vi "Keysight E36300 Series Run Data Logger.vi"() -> ()   [LabVIEW 2020]
doc: "This example runs data logger.\n\nNote:\nThis VI is only available on the E36312A and E36313A models."
uses:
  Keysight E36300 Series.lvlib
panel:
  in  "Channel (1)":string="1"
  out "Logged Data":dbl[](array[numeric])
  in  "Reading Count (0)":i32
  in  "Trigger Source (0: Bus)":i32(ring) items=["Bus", "External", "Immediate"]
  in  "Sample Interval (0.2 sec)":dbl=0.2
  in  "Sample Duration (1 sec)":dbl=1.0
  in  "Enable Extremum (T: Enable)":bool=TRUE
  in  "Enable Data Logging (T: Enable)":bool=TRUE
  in  "Data Logging (0: Current)":i32(ring) items=["Current", "Voltage"]
  in  "Data Save Path(\"External:\\log_1.csv\")":string="\"External:\\log_1.csv\""
  in  "VISA resource name":refnum<visa-resource-name>
  # "(c) 2019 - 2021 National Instruments.  ALL RIGHTS RESERVED."
  # "This VI is only available on the E36312A and E36313A models."
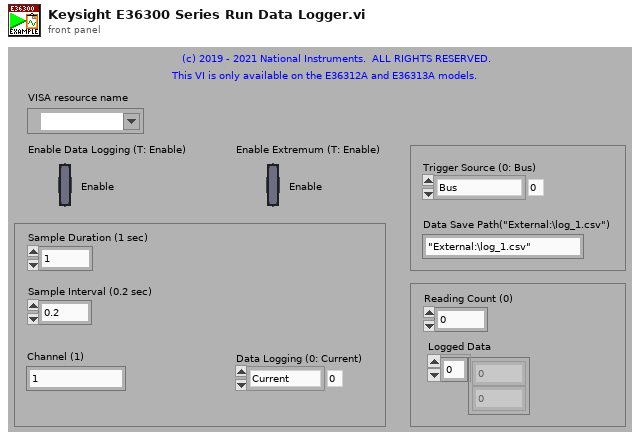
[diagram p1: front panel]
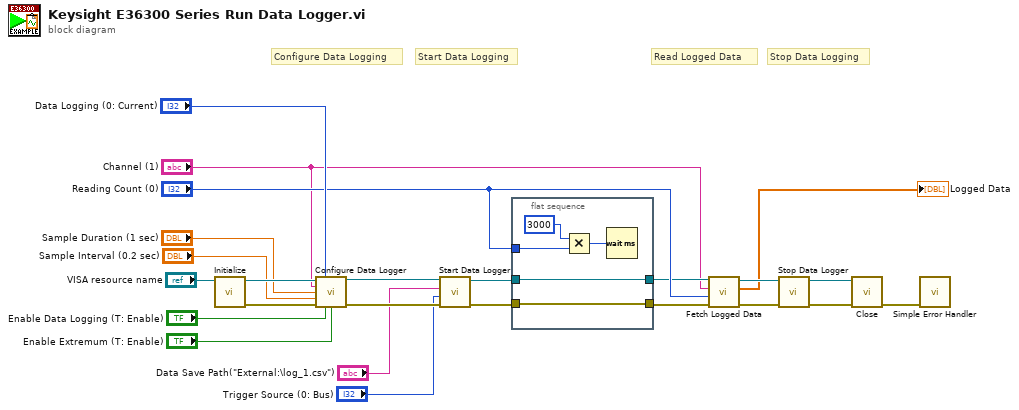
[diagram p0: block diagram]
diagram:
  # "Read Logged Data"
  # "Stop Data Logging"
  # "Start Data Logging"
  # "Configure Data Logging"
  n1 = call "Initialize.vi"("VISA resource name"="VISA resource name") -> ("error out"=w22:errorcluster, "VISA resource name out"=w23:refnum<visa-resource-name>)  [unwired: 9 in]
  n2 = call "Configure Data Logger.vi"("VISA resource name"=w23, "Data Logging (0: Current)"="Data Logging (0: Current)", "Channel (1)"="Channel (1)", "Sample Duration (1 sec)"="Sample Duration (1 sec)", "Sample Interval (0.2 sec)"="Sample Interval (0.2 sec)", "error in (no error)"=w22, "Enable Data Logging (T: Enable)"="Enable Data Logging (T: Enable)", "Enable Extremum (T: Enable)"="Enable Extremum (T: Enable)") -> ("VISA resource name out"=w4:refnum<visa-resource-name>, "error out"=w5:errorcluster)  [unwired: 6 in]
  n3 = call "Start Data Logger.vi"("error in (no error)"=w5, "Trigger Source (0: Bus)"="Trigger Source (0: Bus)", "Data Save Path (\"External:\\log_1.csv\")"="Data Save Path(\"External:\\log_1.csv\")", "VISA resource name"=w4) -> ("error out"=w6:errorcluster, "VISA resource name out"=w7:refnum<visa-resource-name>)  [unwired: 6 in]
  n4 = flat-sequence {
    tunnel: "Reading Count (0)" -> [w29]
    tunnel: w7 -> [w26]
    tunnel: [w26] -> w8
    tunnel: w6 -> [w25]
    tunnel: [w25] -> w10
    frame #0 {
      n5 = Multiply(x=3000, y=w29) -> (x*y=w27:i32)
      n6 = Wait (ms)(milliseconds to wait=w27) -> ()  [unwired: 1 out]
    }
  }
  n7 = call "Fetch Logged Data.vi"("error in (no error)"=w10, "Reading Count (0)"="Reading Count (0)", "Channel (1)"="Channel (1)", "VISA resource name"=w8) -> ("error out"=w12:errorcluster, "Logged Data"=→"Logged Data":dbl[], "VISA resource name out"=w13:refnum<visa-resource-name>)  [unwired: 5 in]
  n8 = call "Stop Data Logger.vi"("error in (no error)"=w12, "VISA resource name"=w13) -> ("error out"=w14:errorcluster, "VISA resource name out"=w15:refnum<visa-resource-name>)  [unwired: 8 in]
  n9 = call "Close.vi"("error in (no error)"=w14, "VISA resource name"=w15) -> ("error out"=w16:errorcluster)  [unwired: 9 in]
  n10 = call <vilib>:"Simple Error Handler.vi"("error in (no error)"=w16) -> ()  [unwired: 4 in, 5 out]
